vi "Initialize Camera.vi"(8 "error in (no error)":errorcluster, 11 "CCDCamera in":refnum<class "Real Camera.lvclass">) -> (0 "error out":errorcluster, 3 "CCDCamera out":refnum<class "Real Camera.lvclass">)   [LabVIEW 2018, in "Real Camera.lvclass"]
doc: "Initialize the camera\n\nBefore initializing the camera, this function tests if the connect camera is an iXon Ultra. If so, it continues with the execution. Otherwise, it will do a shut down and pass to the next camera (if applicable)."
uses:
  Real Camera.lvclass
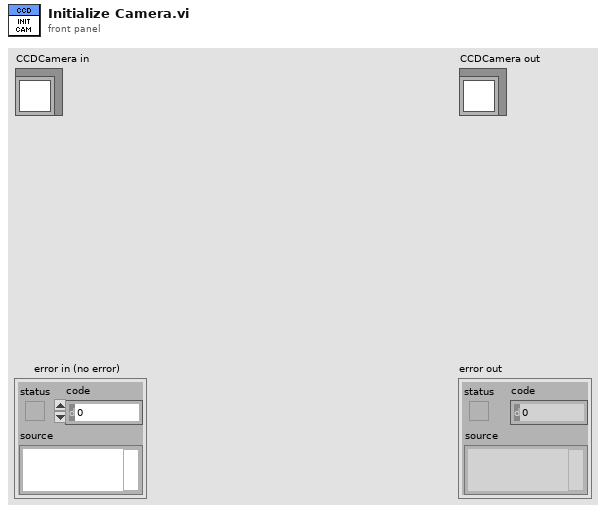
[diagram p1: front panel]
types:
  T1 = typedef "AndorCapabilities typedef.ctl" = cluster{"AcqModes":cluster{"single":bool, "video":bool, "accumulate":bool, "kinetic":bool, "frametransfer":bool, "fastkinetics":bool}, "ReadModes":cluster{"fullimage":bool, "subimage":bool, "singletrack":bool, "fvb":bool, "multitrack":bool, "randomtrack":bool}, "TriggerModes":cluster{"internal":bool, "external":bool}, "CameraType":enum32{"PDA", "iXon", "ICCD", "EMCCD", "CCD", "iStar", "third party camera", "iDus", "Newton", "Surcam", "USB ICCD", "Luca", "Reserved", "iKon", "InGaAs", "iVac", "Unprogrammed", "Clara", "USB iStar", "SimCam", "Neo", "iXon Ultra", "Volmos", "iVac Ultra"}, "PixelMode":cluster{"8-bit":bool, "14-bit":bool, "16-bit":bool, "32-bit":bool, "color mode":enum16{"Mono", "RGB", "CMY"}}, "SetFunctions":cluster{"vreadout":bool, "hreadout":bool, "temperature":bool, "gain":bool, "emccdgain":bool}, "GetFunctions":cluster{"temperature":bool, "targettemperature":bool, "temperaturerange":bool, "detectorsize":bool, "gain":bool, "emccdgain":bool}, "Features":cluster{"polling":bool, "events":bool, "spooling":bool, "shutter":bool}}
  T2 = enum32{"PDA", "iXon", "ICCD", "EMCCD", "CCD", "iStar", "third party camera", "iDus", "Newton", "Surcam", "USB ICCD", "Luca", "Reserved", "iKon", "InGaAs", "iVac", "Unprogrammed", "Clara", "USB iStar", "SimCam", "Neo", "iXon Ultra", "Volmos", "iVac Ultra"}
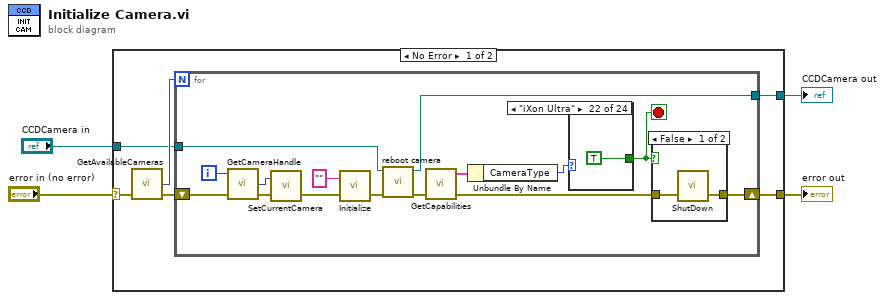
[diagram p0: block diagram]
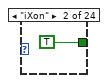
[diagram p4: hidden frame]
diagram:
  n1 = case shown="No Error" "error in (no error)" {
    selector: "error in (no error)" -> [w10 w32]
    tunnel: [w7 w32] -> w1
    tunnel: [w5 w31] -> w2
    tunnel: "CCDCamera in" -> [w6 w31]
    frame No Error {
      n2 = call <userlib>:"GetAvailableCameras.vi"("error in (no error)"=w10) -> ("error out"=w9:errorcluster, "totalCameras"=w8:i32)  [unwired: 2 in, 1 out]
      n3 = for {
        N: w8 -> [_]
        shift-right: [w16] -> w7
        shift-left: w9 -> [w20]
        tunnel: w6 -> [w12]
        tunnel: [w11] -> w5
        i -> [w21]
        stop <- w15 stop-if-true
        n4 = call <userlib>:"GetCameraHandle.vi"("error in (no error)"=w20, "cameraIndex"=w21) -> ("error out"=w22:errorcluster, "cameraHandle"=w18:i32)  [unwired: 1 in, 1 out]
        n5 = call <userlib>:"SetCurrentCamera.vi"("error in (no error)"=w22, "cameraHandle"=w18) -> ("error out"=w19:errorcluster)  [unwired: 1 out]
        n6 = call <userlib>:"Initialize.vi"("error in (no error)"=w19, "directory (\"\")"="" ("directory (\"\")")) -> ("error out"=w14:errorcluster)  [unwired: 1 out]
        n7 = call "reboot camera.vi"("error in (no error)"=w14, "Real Camera in"=w12) -> ("error out"=w13:errorcluster, "Real Camera out"=w11:refnum<class "Real Camera.lvclass">)  [unwired: 8 in]
        n8 = call <userlib>:"GetCapabilities.vi"("error in (no error)"=w13) -> ("error out"=w17:errorcluster, "caps"=w24:T1)  [unwired: 2 in, 1 out]
        n9 = Unbundle By Name(w24) -> ("CameraType"=w23:T2)
        n10 = case shown="\"iXon Ultra\"" w23 {
          tunnel: [_ TRUE _ _ _ _ _ _ _ _ _ _ _ _ _ _ _ _ _ _ _ TRUE _ _] -> w15
          frame "PDA", Default {
          }
          frame "iXon" {
          }
          frame "ICCD" {
          }
          frame "EMCCD" {
          }
          frame "CCD" {
          }
          frame "iStar" {
          }
          frame "third party camera" {
          }
          frame "iDus" {
          }
          frame "Newton" {
          }
          frame "Surcam" {
          }
          frame "USB ICCD" {
          }
          frame "Luca" {
          }
          frame "Reserved" {
          }
          frame "iKon" {
          }
          frame "InGaAs" {
          }
          frame "iVac" {
          }
          frame "Unprogrammed" {
          }
          frame "Clara" {
          }
          frame "USB iStar" {
          }
          frame "SimCam" {
          }
          frame "Neo" {
          }
          frame "iXon Ultra" {
          }
          frame "Volmos" {
          }
          frame "iVac Ultra" {
          }
        }
        n11 = case shown="False" w15 {
          tunnel: w17 -> [w27 w28]
          tunnel: [w26 w28] -> w16
          frame False {
            n12 = call <userlib>:"ShutDown.vi"("error in (no error)"=w27) -> ("error out"=w26:errorcluster)  [unwired: 1 in, 1 out]
          }
          frame True {
          }
        }
      }
    }
    frame Error {
    }
  }
  "error out" <- w1
  "CCDCamera out" <- w2
